vi "SlipControl.vi"(10 "Input Cluster":T3 {"Back Right Current" step=0.1; "Front Right Current" step=0.1; "Back Left Current" step=0.1; "Front Left Current" step=0.1}) -> (2 "Output Cluster":T2)   [LabVIEW 2020]
uses:
  SlipControlStates.ctl
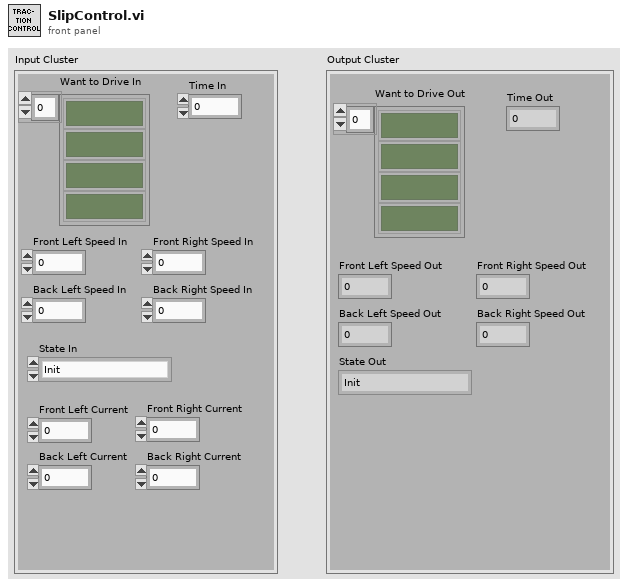
[diagram p1: front panel]
types:
  T1 = typedef "SlipControlStates.ctl" = enum16{"Init", "Grab Time", "Wait", "Grab Time (good)", "Waiting (while run)", "Check", "Grab Time (bad)", "Wait (No Run)"}
  T2 = cluster{"Want to Drive Out":bool[], "Time Out":dbl, "Front Left Speed Out":dbl, "Back Left Speed Out":dbl, "Front Right Speed Out":dbl, "Back Right Speed Out":dbl, "State Out":T1}
  T3 = cluster{"Want to Drive In":bool[], "Time In":dbl, "Front Left Speed In":dbl, "Back Left Speed In":dbl, "Front Right Speed In":dbl, "Back Right Speed In":dbl, "State In":T1, "Front Left Current":dbl, "Back Left Current":dbl, "Front Right Current":dbl, "Back Right Current":dbl}
  T4 = cluster{"Want to Drive In[0]":bool, "Want to Drive In[1]":bool, "Want to Drive In[2]":bool, "Want to Drive In[3]":bool, "Want to Drive In[4]":bool, "Want to Drive In[5]":bool, "Want to Drive In[6]":bool, "Want to Drive In[7]":bool, "Want to Drive In[8]":bool}
  T5 = cluster{"Want to Drive In":bool[], "Time In":dbl, "Front Left Speed In":dbl, "Back Left Speed In":dbl, "Front Right Speed In":dbl, "Back Right Speed In":dbl, T1}
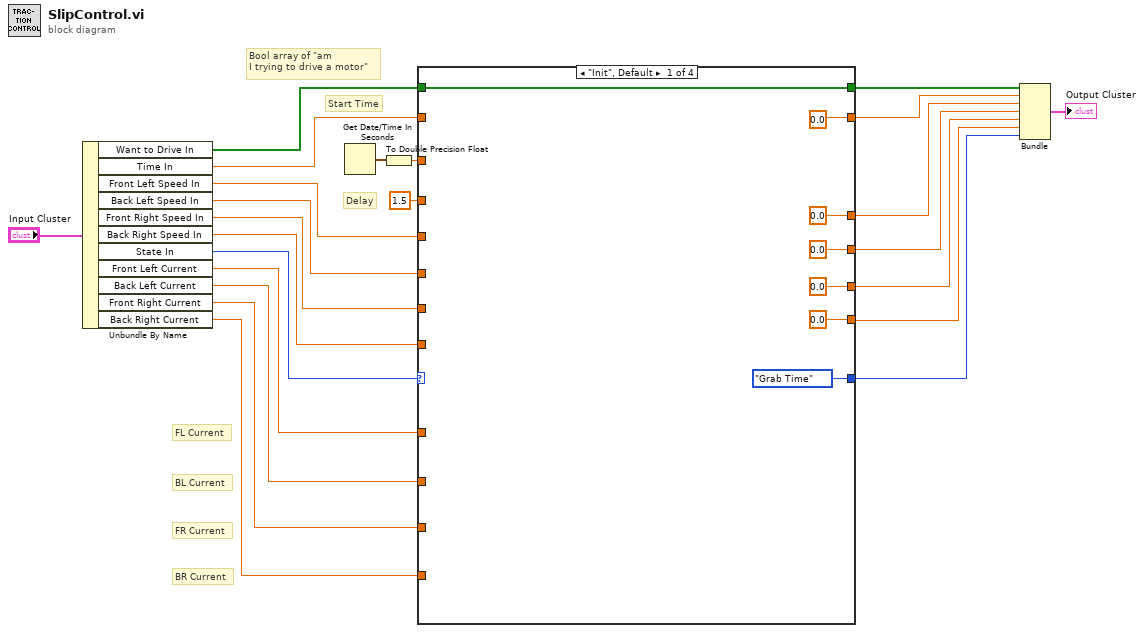
[diagram p0: block diagram]
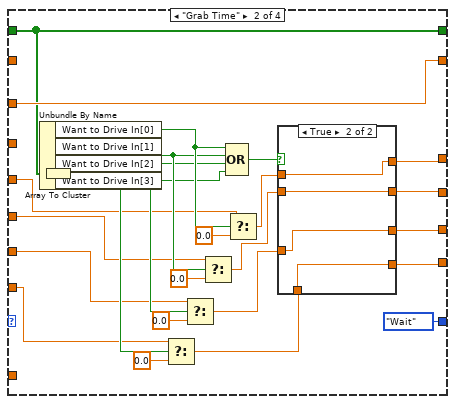
[diagram p2: hidden frame]
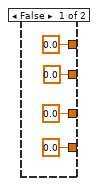
[diagram p3: hidden frame]
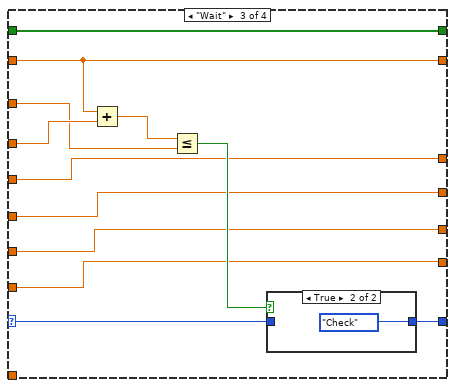
[diagram p4: hidden frame]
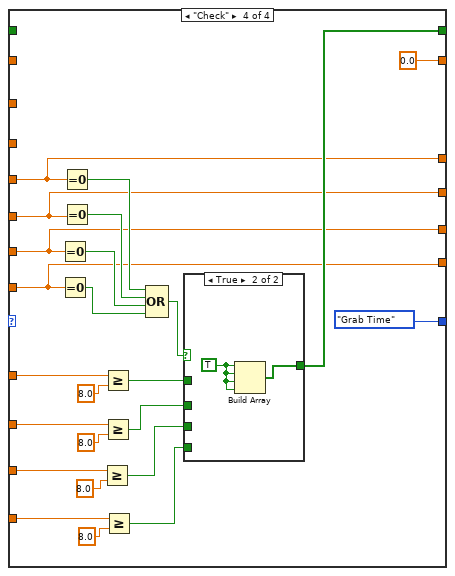
[diagram p6: hidden frame]
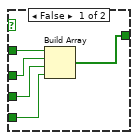
[diagram p7: hidden frame]
diagram:
  # "Delay"
  # "Bool array of \"am \nI trying to drive a motor\""
  # "BR Current"
  # "FR Current"
  # "BL Current"
  # "FL Current"
  # "Start Time"
  n1 = Unbundle By Name("Input Cluster") -> ("Want to Drive In"=w20:bool[], "Time In"=w19:dbl, "Front Left Speed In"=w17:dbl, "Back Left Speed In"=w16:dbl, "Front Right Speed In"=w15:dbl, "Back Right Speed In"=w14:dbl, "State In"=w13:T1, "Front Left Current"=w12:dbl, "Back Left Current"=w11:dbl, "Front Right Current"=w10:dbl, "Back Right Current"=w9:dbl)
  n2 = Get Date/Time In Seconds() -> (seconds since 1Jan1904=w23:timestamp)
  n3 = To Double Precision Float(number=w23) -> (double precision float=w22:dbl)
  n4 = case shown="\"Init\", Default" w13 {
    selector: w13 -> [_ _ w68 _]
    tunnel: [0.0 w54 w67 w81] -> w5
    tunnel: [SlipControlStates."Grab Time" SlipControlStates."Wait" w69 SlipControlStates."Grab Time"] -> w1
    tunnel: w22 -> [_ w55 w71 _]
    tunnel: [0.0 w55 w74 0.0] -> w6
    tunnel: w19 -> [_ _ w74 _]
    tunnel: 1.5 ("Delay") -> [_ _ w73 _]
    tunnel: w12 -> [_ _ _ w85]
    tunnel: w11 -> [_ _ _ w84]
    tunnel: [w27 w49 w75 w97] -> w8
    tunnel: w20 -> [w27 w49 w75 _]
    tunnel: w10 -> [_ _ _ w83]
    tunnel: w9 -> [_ _ _ w82]
    tunnel: [0.0 ("Back Left Speed") w52 w66 w80] -> w4
    tunnel: [0.0 ("Front Right Speed") w51 w65 w79] -> w3
    tunnel: [0.0 ("Back Right Speed") w50 w64 w78] -> w2
    tunnel: w17 -> [_ w34 w67 w81]
    tunnel: w16 -> [_ w33 w66 w80]
    tunnel: w15 -> [_ w32 w65 w79]
    tunnel: w14 -> [_ w31 w64 w78]
    frame "Init", Default {
    }
    frame "Grab Time" {
      n5 = Array To Cluster(array=w49) -> (cluster=w48:T4)
      n6 = Unbundle By Name(w48) -> ("Want to Drive In[0]"=w46:bool, "Want to Drive In[1]"=w43:bool, "Want to Drive In[2]"=w41:bool, "Want to Drive In[3]"=w39:bool)
      n7 = Select(t=w31, s=w39, f=0.0) -> (s? t:f=w35:dbl)
      n8 = Select(t=w32, s=w41, f=0.0) -> (s? t:f=w36:dbl)
      n9 = Select(t=w33, s=w43, f=0.0) -> (s? t:f=w37:dbl)
      n10 = Compound Arithmetic op=OR(w46, w43, w41, w39) -> (w47:bool)
      n11 = Select(t=w34, s=w46, f=0.0) -> (s? t:f=w38:dbl)
      n12 = case shown="True" w47 {
        tunnel: [0.0 w63] -> w54
        tunnel: [0.0 ("Back Left Speed") w62] -> w52
        tunnel: [0.0 ("Front Right Speed") w60] -> w51
        tunnel: [0.0 ("Back Right Speed") w61] -> w50
        tunnel: w38 -> [_ w63]
        tunnel: w37 -> [_ w62]
        tunnel: w36 -> [_ w60]
        tunnel: w35 -> [_ w61]
        frame False {
        }
        frame True {
        }
      }
    }
    frame "Wait" {
      n13 = Add(x=w74, y=w73) -> (x+y=w72:dbl)
      n14 = Less Or Equal?(x=w72, y=w71) -> (x <= y?=w70:bool)
      n15 = case shown="True" w70 {
        tunnel: [w76 SlipControlStates."Check"] -> w69
        tunnel: w68 -> [w76 _]
        frame False {
        }
        frame True {
        }
      }
    }
    frame "Check" {
      n16 = Equal To 0?(x=w79) -> (x = 0?=w88:bool)
      n17 = Equal To 0?(x=w78) -> (x = 0?=w87:bool)
      n18 = Equal To 0?(x=w81) -> (x = 0?=w90:bool)
      n19 = Equal To 0?(x=w80) -> (x = 0?=w89:bool)
      n20 = Greater Or Equal?(x=w83, y=8.0) -> (x >= y?=w92:bool)
      n21 = Greater Or Equal?(x=w85, y=8.0) -> (x >= y?=w98:bool)
      n22 = Greater Or Equal?(x=w84, y=8.0) -> (x >= y?=w93:bool)
      n23 = Greater Or Equal?(x=w82, y=8.0) -> (x >= y?=w91:bool)
      n24 = Compound Arithmetic op=OR(w90, w89, w88, w87) -> (w86:bool)
      n25 = case shown="True" w86 {
        tunnel: w98 -> [w106 _]
        tunnel: [w102 w107] -> w97
        tunnel: w93 -> [w105 _]
        tunnel: w92 -> [w104 _]
        tunnel: w91 -> [w103 _]
        frame False {
          n26 = Build Array(w106, w105, w104, w103) -> (w102:bool[])
        }
        frame True {
          w108 = TRUE
          n27 = Build Array(w108, w108, w108, w108) -> (w107:bool[])
        }
      }
    }
  }
  n28 = Bundle("Want to Drive In"=w8, "Time In"=w6, "Front Left Speed In"=w5, "Back Left Speed In"=w4, "Front Right Speed In"=w3, "Back Right Speed In"=w2, w1) -> (→"Output Cluster":T5)  [unwired: 1 in]
